vi "AddTaskDataConfiguration.vi"(6 "argument":i32, 8 "error in (no error)":errorcluster, 9 "task data signal":u32(ring)=106 items=["ActiveFixtureOffset"=106, "ActiveMoveValid"=435, "AxesSlowdownReason"=448, "CannedFunctionID"=240, "CoordinatedAccelerationCommand"=64, "CoordinatedAccelerationRate"=132, "CoordinatedAccelerationTime"=134, "CoordinatedArcEndAngle"=59, "CoordinatedArcRadius"=60, "CoordinatedArcRadiusError"=61, "CoordinatedArcRadiusReciprocal"=363, "CoordinatedArcStartAngle"=58, "CoordinatedDecelerationRate"=133, "CoordinatedDecelerationTime"=135, "CoordinatedFlags"=45, "CoordinatedGalvoLaserOutput"=169, "CoordinatedMotionRate"=184, "CoordinatedPercentDone"=66, "CoordinatedPositionCommand"=62, "CoordinatedPositionCommandBackwardsDiff"=67, "CoordinatedSpeedCommand"=63, "CoordinatedSpeedTarget"=124, "CoordinatedSpeedTargetActual"=104, "CoordinatedTaskCommand"=185, "CoordinatedTimeScale"=370, "CoordinatedTimeScaleDerivative"=371, "CoordinatedTotalDistance"=65, "CoordinateSystem1I"=118, "CoordinateSystem1J"=119, "CoordinateSystem1K"=120, "CoordinateSystem1Plane"=121, "CriticalSectionActive"=440, "DependentCoordinatedSpeedTarget"=125, "DependentCoordinatedSpeedTargetActual"=105, "EnableAlignmentAxes"=159, "EnableState"=224, "ExecutionMode"=151, "FiberMoveCount"=195, "FiberPower"=273, "FiberPowerOptimal"=274, "FiberPowerSampleCount"=275, "FiberSearchResult"=276, "IFOVAttemptCode"=394, "IFOVCenterPointH"=390, "IFOVCenterPointV"=391, "IFOVCoordinatedAccelerationCommand"=399, "IFOVCoordinatedPositionCommand"=385, "IFOVCoordinatedSpeedCommand"=386, "IFOVFOVDimensionH"=402, "IFOVFOVDimensionV"=403, "IFOVFOVPositionH"=400, "IFOVFOVPositionV"=401, "IFOVGenerationFrameCounter"=382, "IFOVGenerationFrameIndex"=395, "IFOVGenerationTimeModified"=384, "IFOVGenerationTimeOriginal"=383, "IFOVIdealVelocity"=397, "IFOVMaximumVelocity"=396, "IFOVSpeedScale"=380, "IFOVSpeedScaleAverage"=381, "IFOVTrajectoryCount"=392, "IFOVTrajectoryIndex"=393, "ImmediateCommandErrorCode"=329, "ImmediateCommandErrorLocation"=330, "ImmediateState"=155, "LookaheadMovesExamined"=278, "MFO"=123, "MotionBufferElements"=427, "MotionBufferIndex"=432, "MotionBufferIndexLookahead"=433, "MotionBufferMoves"=428, "MotionBufferProcessingBlocked"=434, "MotionBufferRetraceElements"=431, "MotionBufferRetraceMoves"=430, "MotionEngineStage"=367, "MotionLineNumber"=429, "ProfileControlMask"=324, "ProgramLineNumber"=17, "ProgramLineNumberInternal"=322, "ProgramPersistent"=154, "ProgramVariable"=75, "QueueLineCapacity"=326, "QueueLineCount"=325, "QueueStatus"=162, "SchedulerProgramLoopRuns"=438, "SchedulerTaskBlocked"=439, "SchedulerTaskHolds"=437, "Spindle0SpeedTarget"=112, "Spindle1SpeedTarget"=113, "Spindle2SpeedTarget"=114, "Spindle3SpeedTarget"=115, "TaskDoubleVariable"=248, "TaskErrorCode"=79, "TaskErrorLocation"=152, "TaskExecutionLines"=436, "TaskExecutionLinesMaximum"=452, "TaskExecutionTime"=450, "TaskExecutionTimeMaximum"=451, "TaskInfoVariable"=249, "TaskInternalDebug"=398, "TaskMode"=137, "TaskParameter"=77, "TaskReturnVariable"=271, "TaskState"=146, "TaskStateInternal"=147, "TaskStatus0"=108, "TaskStatus1"=109, "TaskStatus2"=110, "TaskWarningCode"=80, "TaskWarningLocation"=153, "ToolNumberActive"=122, "WaitCommandDuration"=103], 10 "taskId in":i32(ring) items=["TLibrary", "T01", "T02", "T03", "T04", "T05", "T06", "T07", "T08", "T09", "T10", "T11", "T12", "T13", "T14", "T15", "T16", "T17", "T18", "T19", "T20", "T21", "T22", "T23", "T24", "T25", "T26", "T27", "T28", "T29", "T30", "T31"], 11 "controller in":refnum<k24>) -> (0 "error out":errorcluster, 2 "taskId out":i32(ring) items=["TLibrary", "T01", "T02", "T03", "T04", "T05", "T06", "T07", "T08", "T09", "T10", "T11", "T12", "T13", "T14", "T15", "T16", "T17", "T18", "T19", "T20", "T21", "T22", "T23", "T24", "T25", "T26", "T27", "T28", "T29", "T30", "T31"], 3 "controller out":refnum<k24>)   [LabVIEW 2010]
uses:
  c:/aerotech/controller/stable/A3200/pc/labview/2010/bin/Aerotech.A3200.dll
  bin/Aerotech.A3200.dll
  c:/aerotech/controller/stable/A3200/pc/labview/2010/bin/Aerotech.A3200.LabVIEW.dll
  bin/Aerotech.A3200.LabVIEW.dll
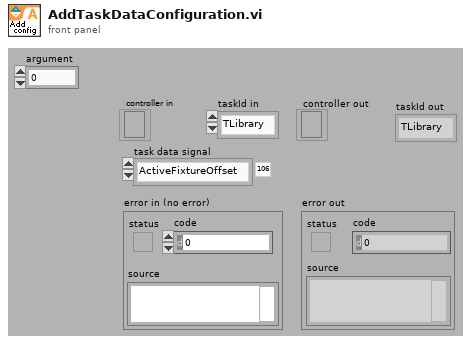
[diagram p1: front panel]
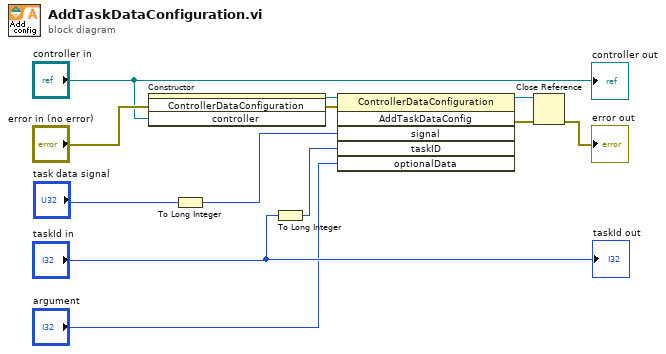
[diagram p0: block diagram]
diagram:
  n1 = constructor class="ControllerDataConfiguration"(error in="error in (no error)", "controller"="controller in") -> (reference out=w11:refnum<k24>, error out=w10:errorcluster)  [unwired: 2 in, 2 out]
  n2 = To Long Integer(number="task data signal") -> (32bit integer=w4:i32)
  n3 = To Long Integer(number="taskId in") -> (32bit integer=w3:i32)
  n4 = invoke class="ControllerDataConfiguration" method="AddTaskDataConfig"(reference=w11, error in=w10, "signal"=w4, "taskID"=w3, "optionalData"="argument") -> (reference out=w8:refnum<k24>, error out=w7:errorcluster)  [unwired: 1 in, 4 out]
  n5 = Close Reference(reference=w8, error in (no error)=w7) -> (error out=→"error out":errorcluster)
  "controller out" <- "controller in"
  "taskId out" <- "taskId in"
